vi "Lookup Qs for Type.vi"(8 "error in (no error)":errorcluster, 10 "Identity - Type Only":refnum<class "Identity.lvclass">, 11 "VolatusAPI in":refnum<class "VolatusAPI.lvclass">) -> (0 "error out":errorcluster, 2 "MessageQs":refnum<class "MessageQ.lvclass">[](array[class]), 3 "VolatusAPI out":refnum<class "VolatusAPI.lvclass">)   [LabVIEW 2020, in "Volatus.lvlib" / "VolatusAPI.lvclass"]
uses:
  VolatusAPI.lvclass
  Identity/Identity.lvclass
  MessageQ/MessageQ.lvclass
  VolatusAPI.lvclass/VolatusAPI.ctl
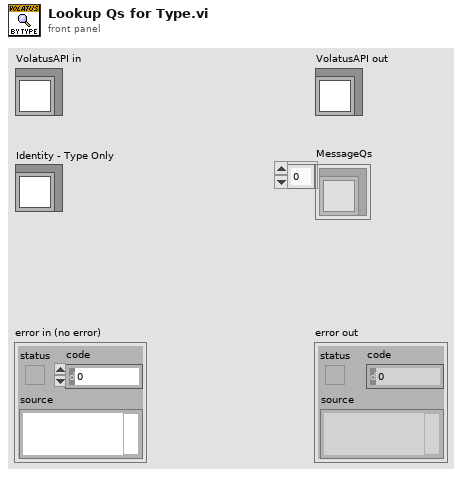
[diagram p1: front panel]
types:
  T1 = typedef "Volatus.lvlib/VolatusAPI.lvclass/MsgQs Ref.ctl" = cluster{"Keys":map{string, T2}, "MsgQs":map{i32, T3}, "Next Number":i32}
  T2 = typedef "Volatus.lvlib/VolatusAPI.lvclass/Q Info.ctl" = cluster{"Number":i32, "Notifiers":refnum<notifier>[]}
  T3 = typedef "Volatus.lvlib/VolatusAPI.lvclass/Registered Q.ctl" = cluster{"Q":refnum<class "MessageQ.lvclass">, "Keys":string[]}
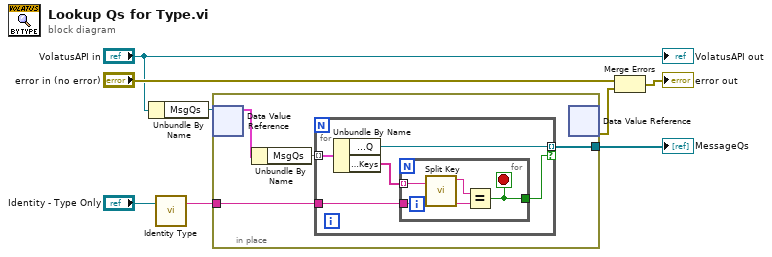
[diagram p0: block diagram]
diagram:
  n1 = Unbundle By Name("VolatusAPI in") -> ("MsgQs"=w7:refnum<data-value>)
  n2 = call-dynamic "Identity Type.vi"("Identity in"="Identity - Type Only") -> ("Type"=w4:string)  [unwired: 2 in]
  n3 = in-place {
    in-place-border: w4 -> [w10]
    in-place-border: [w9] -> w3
    n4 = in-place-dvr #1(w7) -> (w12:T1)  [unwired: 1 out]
    n5 = Unbundle By Name(w12) -> ("MsgQs"=w11:map{i32, T3})
    n6 = for {
      tunnel: w11 -> [w17] mode=indexing
      tunnel: w10 -> [w15]
      tunnel: [w14] -> w9 mode=indexing if=w13
      n7 = Unbundle By Name(w17) -> ("Registered API.Q"=w14:refnum<class "MessageQ.lvclass">, "Registered API.Keys"=w16:string[])
      n8 = for {
        tunnel: w16 -> [w21] mode=indexing
        tunnel: w15 -> [w19]
        tunnel: [w18] -> w13
        stop <- w18 stop-if-true
        n9 = call "Split Key.vi"("Key"=w21) -> ("Type"=w20:string)  [unwired: 3 in, 1 out]
        n10 = Equal?(x=w20, y=w19) -> (x = y?=w18:bool)
      }
    }
    n11 = in-place-dvr #1() -> (w1:errorcluster)  [unwired: 1 in, 1 out]
  }
  "MessageQs" <- w3
  n12 = Merge Errors("error in (no error)", w1) -> (→"error out":errorcluster)
  "VolatusAPI out" <- "VolatusAPI in"
